vi "Starting Square Type.vi"(11 "Team in":refnum<class "Team.lvclass">) -> (2 "Square":refnum<class "Square.lvclass">, 3 "Team out":refnum<class "Team.lvclass">)   [LabVIEW 2020, in "SquareBattle.lvlib" / "Team.lvclass"]
doc: "Determines the square class that should be placed as the first square for a team."
uses:
  Team.lvclass
  Square/Square.lvclass
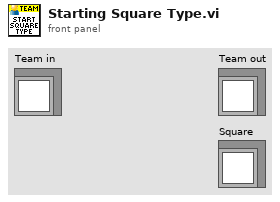
[diagram p1: front panel]
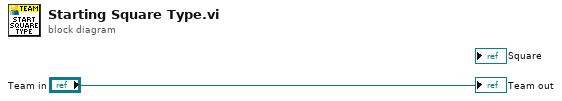
[diagram p0: block diagram]
diagram:
  "Team out" <- "Team in"
